vi "SavePupilCameraImages.vi"(5 "Save Format":enum16{"Png", "Raw"}(ring), 7 "Save Image?":bool, 8 "Block Folder":path, 9 "Subfolder":string="Eyetracker", 10 "Refnum in":T1) -> (2 "Refnum out (duplicate)":T1, 3 "ImageSaved":bool=TRUE)   [LabVIEW 2017]
uses:
  <vilib>/vision/Image Controls.llb/IMAQ Image.ctl
  <vilib>/Utility/file.llb/Write To Spreadsheet File (string).vi
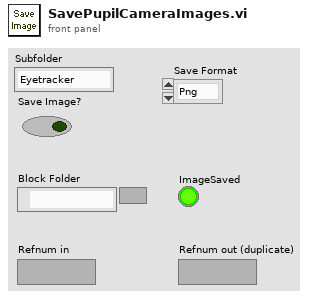
[diagram p1: front panel]
types:
  T1 = typedef "IMAQ Image.ctl" = refnum<image>
  T2 = enum16{"open", "replace", "create", "open or create", "replace or create", "replace or create with confirmation"}
  T3 = cluster{"Desired Font (Application)":enum16{"User-specified Font", "Application Font", "System Font", "Dialog Font"}, "[User-specified Font]":cluster{"Font Name":string, "Size":i16, "Strikeout?":bool, "Italic?":bool, "Underline?":bool, "Outline?":bool, "Shadow?":bool, "Bold?":bool, "Rotation Angle":dbl}, "Horizontal Alignment":i16, "Vertical Alignment":i16}
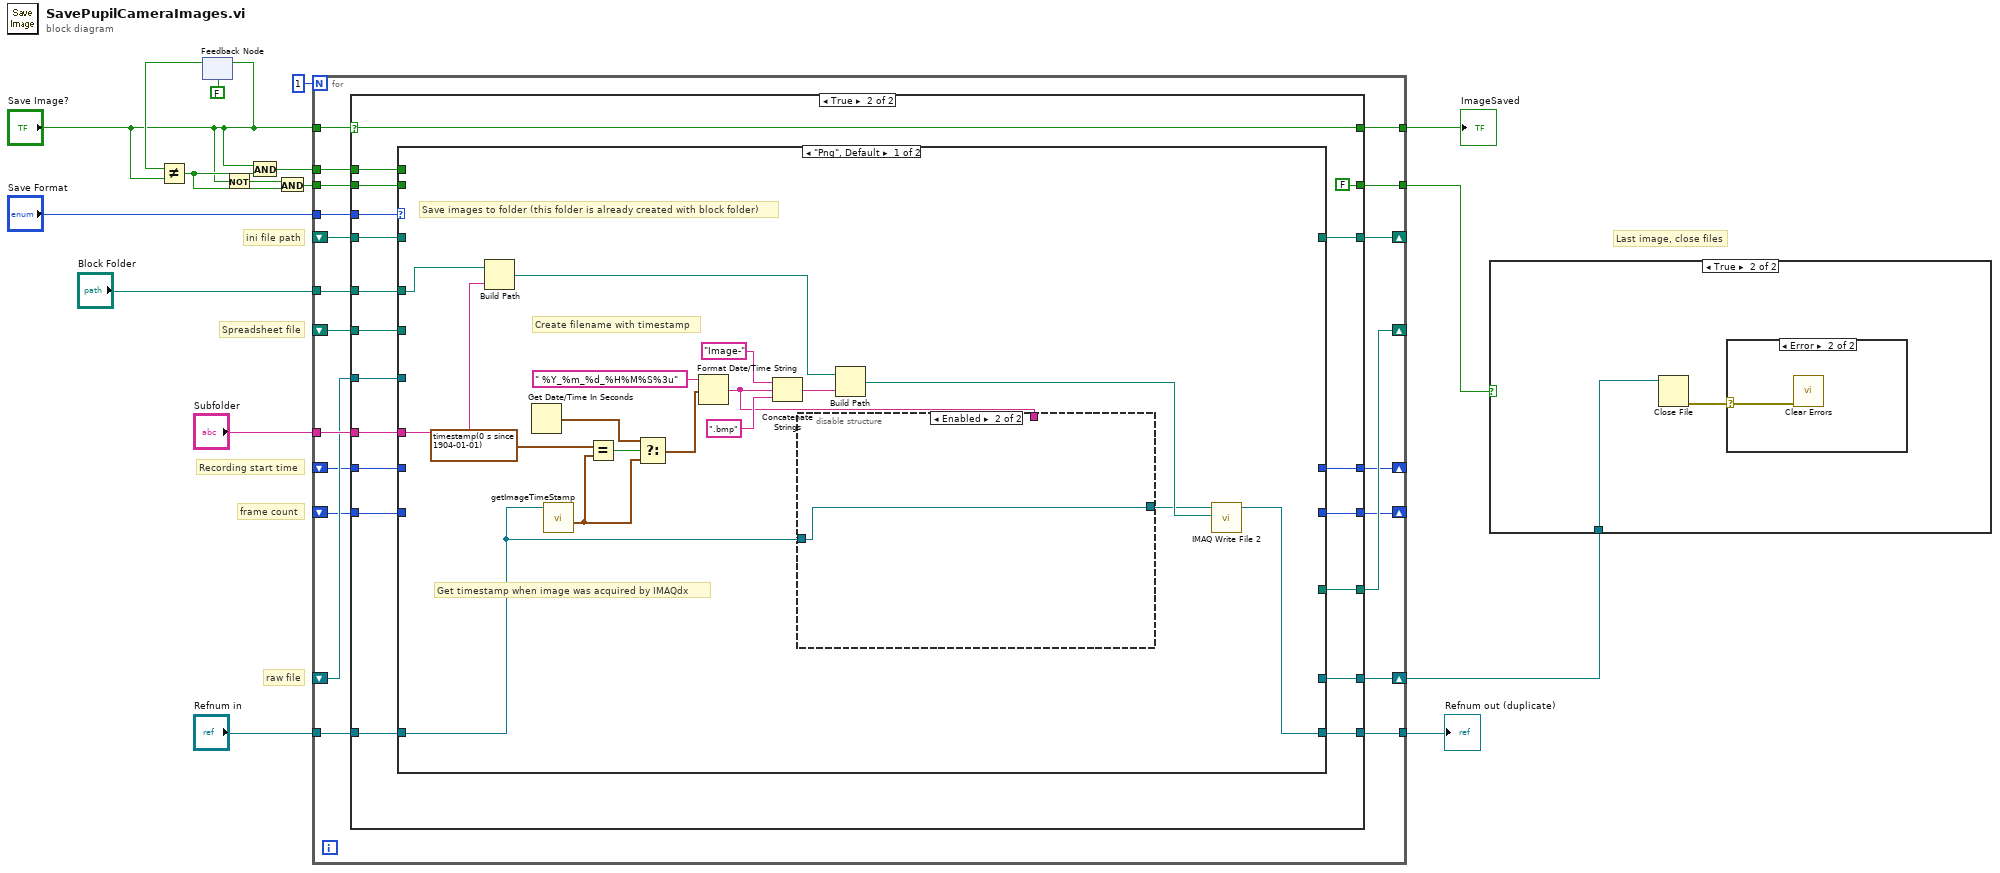
[diagram p0: block diagram]
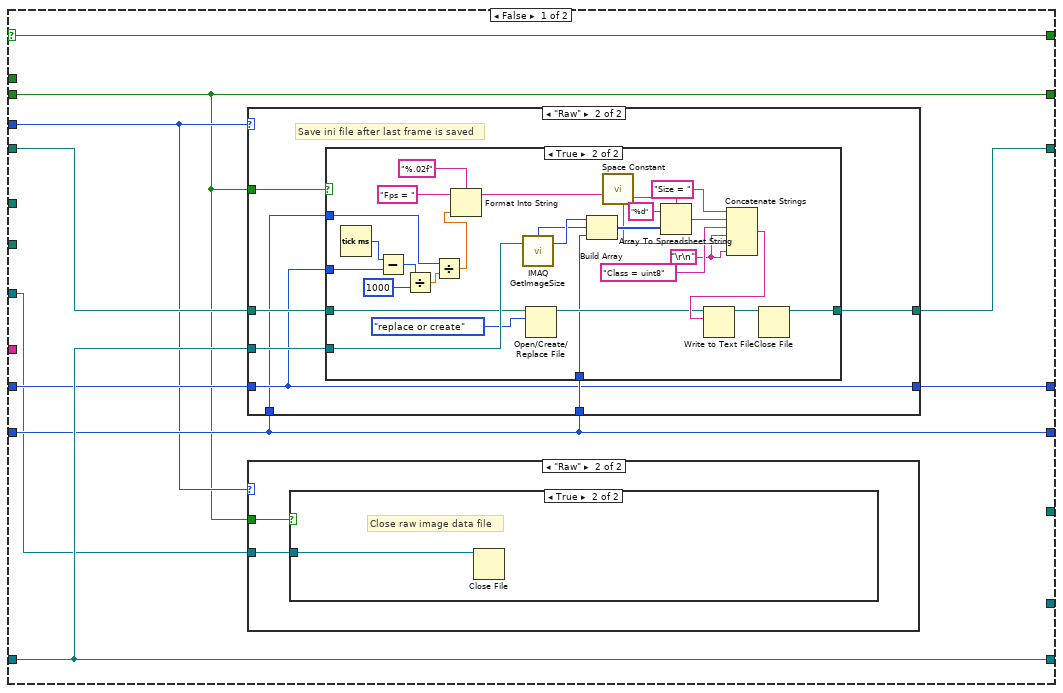
[diagram p4: hidden frame]
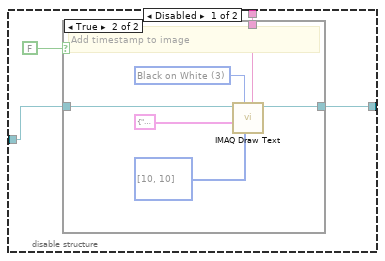
[diagram p9: hidden frame]
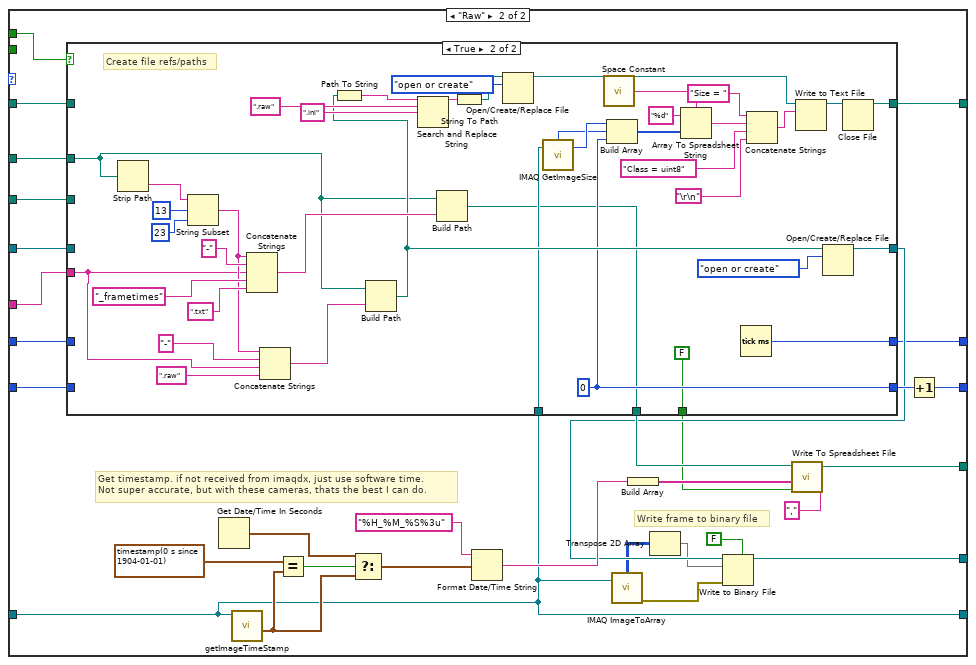
[diagram p11: hidden frame]
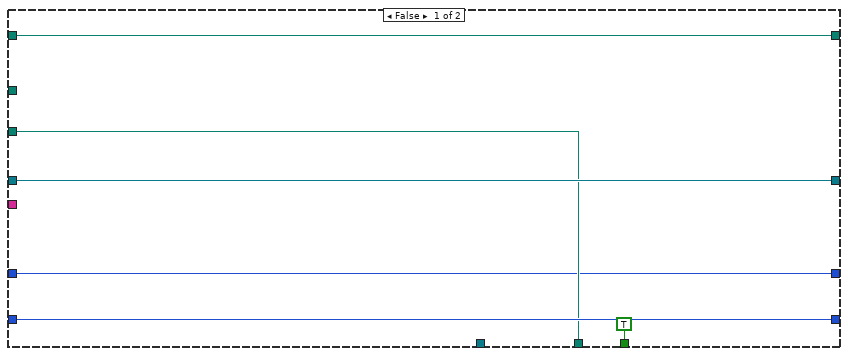
[diagram p12: hidden frame]
diagram:
  # "Recording start time"
  # "frame count"
  # "Spreadsheet file"
  # "raw file"
  # "ini file path"
  # "Last image, close files"
  n1 = feedback-in #1("Save Image?") -> ()
  n2 = feedback #1(FALSE ("Save Image?")) -> (w4:bool)
  n3 = Not Equal?(x=w4, y="Save Image?") -> (x != y?=w3:bool)
  n4 = Not(x="Save Image?") -> (.not. x?=w2:bool)
  n5 = And(x="Save Image?", y=w3) -> (x .and. y?=w6:bool)
  n6 = And(x=w2, y=w3) -> (x .and. y?=w5:bool)
  n7 = for {
    N: 1 -> [_]
    tunnel: [w36] -> w16
    tunnel: "Block Folder" -> [w35]
    tunnel: "Refnum in" -> [w34]
    tunnel: "Save Image?" -> [w33]
    tunnel: [w32] -> w10
    tunnel: "Subfolder" -> [w31]
    tunnel: "Save Format" -> [w30]
    tunnel: w6 -> [w29]
    shift-right: [w28] -> _
    shift-left: _ -> [w27]
    shift-right: [w26] -> w8
    shift-left: _ -> [w25]
    tunnel: w5 -> [w24]
    shift-right: [w23] -> _
    shift-left: _ -> [w22]
    tunnel: [w21] -> w9
    shift-right: [w20] -> _
    shift-left: _ -> [w19]
    shift-right: [w18] -> _
    shift-left: _ -> [w17]
    n8 = case shown="True" w33 {
      selector: w33 -> [w46 w102]
      tunnel: [w45 w104] -> w36
      tunnel: w35 -> [_ w105]
      tunnel: w34 -> [w45 w103]
      tunnel: [w46 w102] -> w32
      tunnel: w31 -> [_ w101]
      tunnel: w30 -> [w39 w100]
      tunnel: w29 -> [_ w99]
      tunnel: [_ w98] -> w26
      tunnel: [_ w97] -> w28
      tunnel: w27 -> [_ w96]
      tunnel: w25 -> [w37 w95]
      tunnel: w24 -> [w38 w94]
      tunnel: [w40 w93] -> w23
      tunnel: w22 -> [w40 w92]
      tunnel: [w38 FALSE ("Last Frame")] -> w21
      tunnel: [w43 w90] -> w20
      tunnel: w19 -> [w44 w89]
      tunnel: [w41 w88] -> w18
      tunnel: w17 -> [w42 w87]
      frame False {
        n9 = case shown="\"Raw\"" w39 {
          tunnel: w45 -> [_ w58]
          tunnel: w40 -> [_ w57]
          tunnel: w44 -> [w51 w56]
          tunnel: [w51 w55] -> w43
          tunnel: w38 -> [_ w54]
          tunnel: w42 -> [w50 w53]
          tunnel: [w50 w53] -> w41
          tunnel: w40 -> [_ w52]
          frame "Png", Default {
          }
          frame "Raw" {
            # "Save ini file after last frame is saved"
            n10 = case shown="True" w54 {
              tunnel: w58 -> [_ w78]
              tunnel: w57 -> [_ w76]
              tunnel: w56 -> [w59 w74]
              tunnel: [w59 w73] -> w55
              tunnel: w53 -> [_ w68]
              tunnel: w52 -> [_ w65]
              frame False {
              }
              frame True {
                w60 = "\r\n"
                n11 = Tick Count (ms)() -> (millisecond timer value=w69:u32)
                n12 = Subtract(x=w69, y=w68) -> (x-y=w67:u32)
                n13 = Divide(x=w67, y=u32 1000) -> (x/y=w64:dbl)
                n14 = Divide(x=w65, y=w64) -> (x/y=w63:dbl)
                n15 = Format Into String(format string="%.02f", initial string="Fps = ", w63) -> (resulting string=w62:string)  [unwired: 1 in, 1 out]
                n16 = call "IMAQ GetImageSize"("Image"=w78) -> ("Y Resolution"=w86:i32, "X Resolution"=w85:i32)  [unwired: 3 in, 1 out]
                n17 = Open/Create/Replace File(file path (use dialog)=w74, operation (0:open)=T2."replace or create") -> (refnum out=w77:refnum<file>)  [unwired: 4 in, 2 out]
                n18 = Build Array(w86, w85, w76) -> (w84:i32[])
                n19 = call <vilib>:"Space Constant.vi"() -> ("String"=w72:string)
                n20 = Array To Spreadsheet String(delimiter (Tab)=w72, array=w84, 3:"%d" ("format string")) -> (spreadsheet string=w82:string)
                n21 = Concatenate Strings("Size = " ("string"), w82, "Class = uint8" ("string"), w60, w62, w60) -> (w79:string)
                n22 = Write to Text File(file (use dialog)=w77, text=w79) -> (refnum out=w80:refnum<file>)  [unwired: 2 in, 2 out]
                n23 = Close File(refnum=w80) -> (path=w73:path)  [unwired: 1 in, 1 out]
              }
            }
          }
        }
        n24 = case shown="\"Raw\"" w39 {
          tunnel: w38 -> [_ w48]
          tunnel: w37 -> [_ w47]
          frame "Png", Default {
          }
          frame "Raw" {
            n25 = case shown="True" w48 {
              tunnel: w47 -> [_ w49]
              frame False {
              }
              frame True {
                # "Close raw image data file"
                n26 = Close File(refnum=w49) -> ()  [unwired: 1 in, 2 out]
              }
            }
          }
        }
      }
      frame True {
        n27 = case shown="\"Png\", Default" w100 {
          tunnel: w105 -> [w117 w152]
          tunnel: [w114 w139] -> w104
          tunnel: w103 -> [w113 w139]
          tunnel: w101 -> [w111 w153]
          tunnel: w99 -> [_ w146]
          tunnel: [_ w154] -> w98
          tunnel: [_ w151] -> w97
          tunnel: w96 -> [_ w150]
          tunnel: w95 -> [_ w149]
          tunnel: w94 -> [_ _]
          tunnel: [_ w147] -> w93
          tunnel: w92 -> [_ w148]
          tunnel: [_ w144] -> w90
          tunnel: w89 -> [_ w142]
          tunnel: [_ w138] -> w88
          tunnel: w87 -> [_ w137]
          frame "Png", Default {
            # "Get timestamp when image was acquired by IMAQdx"
            # "Save images to folder (this folder is already created with block folder)"
            # "Create filename with timestamp"
            n28 = Build Path(base path=w117, name or relative path=w111) -> (appended path=w116:path)
            n29 = Get Date/Time In Seconds() -> (seconds since 1Jan1904=w109:timestamp)
            n30 = call "getImageTimeStamp.vi"("Image refnum in"=w113) -> ("System Time Stamp"=w108:timestamp)  [unwired: 9 in, 1 out]
            n31 = Equal?(x=timestamp(0 s since 1904-01-01), y=w108) -> (x = y?=w110:bool)
            n32 = Select(t=w109, s=w110, f=w108) -> (s? t:f=w107:timestamp)
            n33 = Format Date/Time String(time format string (%c)=" %Y_%m_%d_%H%M%S%3u", seconds (now)=w107) -> (date/time string=w115:string)  [unwired: 1 in]
            n34 = Concatenate Strings("Image-" ("string"), w115, ".bmp" ("string")) -> (w121:string)
            n35 = disable-structure shown="Enabled" {
              disable-tunnel: w115 -> [w126 _]
              disable-tunnel: w113 -> [w124 w134]
              disable-tunnel: [w123 w134] -> w112
              frame Disabled {
                n36 = case shown="True" FALSE {
                  tunnel: w126 -> [_ w133]
                  tunnel: w124 -> [w127 w129]
                  tunnel: [w127 w128] -> w123
                  frame False {
                  }
                  frame True {
                    w130 = 3 items=["White", "Black", "Inverted", "Black on White", "White on Black"] ("Color")
                    # "Add timestamp to image"
                    n37 = call "IMAQ Draw Text"("String"=w133, "Insertion Point"=i32[] [10, 10], "Color"=w130, "Font, Size & Style"=T3 {"Desired Font (Application)"=enum."User-specified Font", "[User-specified Font]"={"Font Name"="", "Size"=26, "Strikeout?"=FALSE, "Italic?"=FALSE, "Underline?"=FALSE, "Outline?"=FALSE, "Shadow?"=FALSE, "Bold?"=FALSE, "Rotation Angle"=0.0}, "Horizontal Alignment"=0, "Vertical Alignment"=1}, "Image Src"=w129) -> ("Image Dst Out"=w128:T1)  [unwired: 3 in, 3 out]
                  }
                }
              }
              frame Enabled {
              }
            }
            n38 = Build Path(base path=w116, name or relative path=w121) -> (appended path=w122:path)
            n39 = call-poly "IMAQ Write File 2"("File Path"=w122, "Image"=w112) -> ("Image Out (duplicate)"=w114:T1)  [unwired: 8 in, 1 out]
          }
          frame "Raw" {
            # "Write frame to binary file"
            # "Get timestamp. if not received from imaqdx, just use software time. \nNot super accurate, but with these cameras, thats the best I can do."
            n40 = case shown="True" w146 {
              tunnel: w153 -> [_ w198]
              tunnel: w152 -> [_ w177]
              tunnel: w150 -> [w169 _]
              tunnel: [w171 w199] -> w141
              tunnel: w149 -> [w171 _]
              tunnel: [w170 w179] -> w145
              tunnel: w148 -> [w170 _]
              tunnel: [w168 w182] -> w144
              tunnel: w139 -> [_ w180]
              tunnel: [w169 w178] -> w143
              tunnel: w142 -> [w168 _]
              tunnel: [TRUE FALSE] -> w140
              tunnel: [w166 w172] -> w138
              tunnel: w137 -> [w166 _]
              frame False {
              }
              frame True {
                w179 = 0
                # "Create file refs/paths"
                n41 = Strip Path(path=w177) -> (name=w207:string)  [unwired: 1 out]
                n42 = String Subset(string=w207, offset (0)=13, length (rest)=23 ("length (rest)")) -> (substring=w202:string)
                n43 = Concatenate Strings(w202, "-" ("string"), w198, "_frametimes" ("string"), ".txt" ("string")) -> (w211:string)
                n44 = Concatenate Strings(w202, "-" ("string"), w198, ".raw" ("string")) -> (w201:string)
                n45 = Build Path(base path=w177, name or relative path=w201) -> (appended path=w193:path)
                n46 = Path To String(path=w193) -> (string=w194:string)
                n47 = Search and Replace String(input string=w194, search string=".raw", replace string=".ini" ("replace string (\"\")")) -> (result string=w197:string)  [unwired: 5 in, 3 out]
                n48 = Build Path(base path=w177, name or relative path=w211) -> (appended path=w178:path)
                n49 = String To Path(string=w197) -> (path=w192:path)
                n50 = Open/Create/Replace File(file path (use dialog)=w192, operation (0:open)=T2."open or create") -> (refnum out=w181:refnum<file>)  [unwired: 4 in, 2 out]
                n51 = call "IMAQ GetImageSize"("Image"=w180) -> ("Y Resolution"=w190:i32, "X Resolution"=w189:i32)  [unwired: 3 in, 1 out]
                n52 = call <vilib>:"Space Constant.vi"() -> ("String"=w175:string)
                n53 = Build Array(w190, w189, w179) -> (w188:i32[])
                n54 = Array To Spreadsheet String(delimiter (Tab)=w175, array=w188, 3:"%d" ("format string")) -> (spreadsheet string=w186:string)
                n55 = Tick Count (ms)() -> (millisecond timer value=w172:u32)
                n56 = Concatenate Strings("Size = " ("string"), w186, "Class = uint8" ("string"), "\r\n") -> (w183:string)
                n57 = Write to Text File(file (use dialog)=w181, text=w183) -> (refnum out=w184:refnum<file>)  [unwired: 2 in, 2 out]
                n58 = Open/Create/Replace File(file path (use dialog)=w193, operation (0:open)=T2."open or create") -> (refnum out=w199:refnum<file>)  [unwired: 4 in, 2 out]
                n59 = Close File(refnum=w184) -> (path=w182:path)  [unwired: 1 in, 1 out]
              }
            }
            n60 = Get Date/Time In Seconds() -> (seconds since 1Jan1904=w163:timestamp)
            n61 = call "getImageTimeStamp.vi"("Image refnum in"=w139) -> ("System Time Stamp"=w160:timestamp)  [unwired: 9 in, 1 out]
            n62 = Equal?(x=timestamp(0 s since 1904-01-01), y=w160) -> (x = y?=w164:bool)
            n63 = Select(t=w163, s=w164, f=w160) -> (s? t:f=w162:timestamp)
            n64 = Format Date/Time String(time format string (%c)="%H_%M_%S%3u", seconds (now)=w162) -> (date/time string=w156:string)  [unwired: 1 in]
            n65 = call "IMAQ ImageToArray"("Image"=w139) -> ("error out"=w158:errorcluster, "Image Pixels (U8)"=w136:u8[][])  [unwired: 3 in, 3 out]
            n66 = Build Array(w156) -> (w155:string[])
            n67 = Transpose 2D Array(2D array=w136) -> (transposed array=w135:u8[][])
            n68 = Write to Binary File(file (use dialog)=w141, data=w135, error in=w158, 5:FALSE ("prepend array or string size? (T)")) -> (refnum out=w154:refnum<file>)  [unwired: 2 in, 2 out]
            n69 = call-poly <vilib>:"Write To Spreadsheet File.vi"("delimiter (\\t)"="," ("delimiter (\\t)"), "append to file? (new file:F)"=w140, "1D data"=w155, "file path (dialog if empty)"=w143) -> ("new file path (Not A Path if cancelled)"=w151:path)  [unwired: 3 in, 1 out]
            n70 = Increment(x=w145) -> (x+1=w147:i32)
          }
        }
      }
    }
  }
  "Refnum out (duplicate)" <- w16
  "ImageSaved" <- w10
  n71 = case shown="True" w9 {
    tunnel: w8 -> [_ w213]
    frame False {
    }
    frame True {
      n72 = Close File(refnum=w213) -> (error out=w212:errorcluster)  [unwired: 1 in, 1 out]
      n73 = case shown="Error" w212 {
        selector: w212 -> [_ w214]
        frame No Error {
        }
        frame Error {
          n74 = call <vilib>:"Clear Errors.vi"("error in (no error)"=w214) -> ()  [unwired: 5 in, 2 out]
        }
      }
    }
  }
